vi "Init.vi"(7 "Prepend Result Name":bool, 8 "error in (no error)":errorcluster, 10 "Measurement Name":string) -> (0 "error out":errorcluster, 3 "SpecAn_IIP3_Calculation out":refnum<class "SpecAn_IIP3_Calculation.lvclass">)   [LabVIEW 2018, in "SeqAuto Evaluations.lvlib" / "SpecAn_IIP3_Calculation.lvclass"]
uses:
  SpecAn_IIP3_Calculation.lvclass
  C:/Sequence Automation/Plugins/SeqAuto IEvaluation.lvlibp/SeqAuto IEvaluation.lvclass
  Plugins/SeqAuto IEvaluation.lvlibp/Write Measurement Name.vi
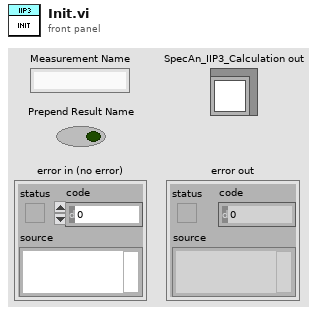
[diagram p1: front panel]
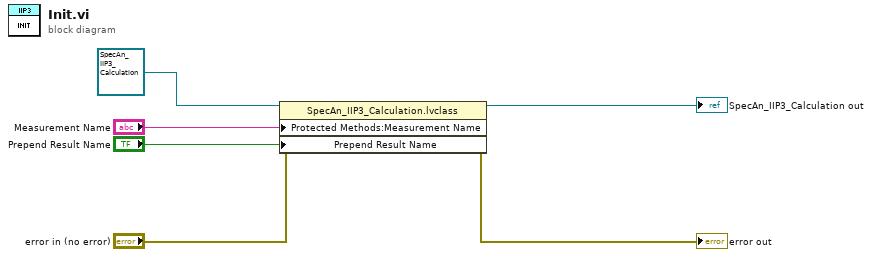
[diagram p0: block diagram]
diagram:
  n1 = property class="SpecAn_IIP3_Calculation.lvclass"(reference=refnum<class "SpecAn_IIP3_Calculation.lvclass"> refnum ("SpecAn_IIP3_Calculation in"), error in="error in (no error)", "Protected Methods:Measurement Name"="Measurement Name", "Prepend Result Name"="Prepend Result Name") -> (reference out=→"SpecAn_IIP3_Calculation out":refnum<class "SpecAn_IIP3_Calculation.lvclass">, error out=→"error out":errorcluster)
